vi "Cache-GEvt Filter Object.vi"() -> (3 "CSM:LogFilter.lvclass":refnum<class "LogFilter.lvclass">)   [LabVIEW 2020, in "Communicable State Machine.lvlib"]
uses:
  Communicable State Machine.lvlib
  LogFilter.lvclass
  global-GEvnt Filter Change Flag.vi
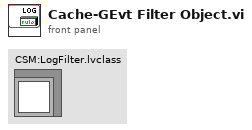
[diagram p1: front panel]
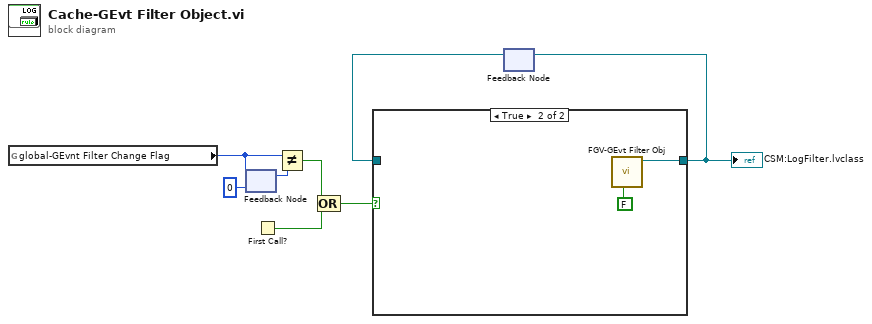
[diagram p0: block diagram]
diagram:
  n1 = global read "global-GEvnt Filter Change Flag.vi" "global-GEvnt Filter Change Flag"() -> (w4:u64)
  n2 = feedback #1(u64 0 ("global-Broadcast Cache Change Flag")) -> (w6:u64)
  n3 = feedback-in #1(w4) -> ()
  n4 = First Call?() -> (First Call?: T/F=w8:bool)
  n5 = Not Equal?(x=w4, y=w6) -> (x != y?=w5:bool)
  n6 = Compound Arithmetic op=OR(w5, w8) -> (w3:bool)
  n7 = feedback #2() -> (w1:refnum<class "LogFilter.lvclass">)  [unwired: 1 in]
  n8 = case shown="True" w3 {
    tunnel: [w9 w10] -> w2
    tunnel: w1 -> [w9 _]
    frame False {
    }
    frame True {
      n9 = call "FGV-GEvt Filter Obj.vi"("Set(T)/Get(F)"=FALSE) -> ("CSM:LogFilter.lvclass"=w10:refnum<class "LogFilter.lvclass">)  [unwired: 9 in, 1 out]
    }
  }
  "CSM:LogFilter.lvclass" <- w2
  n10 = feedback-in #2(w2) -> ()
